vi "Autonomous Independent.vi"   [LabVIEW 2020]
doc: "This VI is called when autonomous begins, and will automatically be terminated when autonomous ends. You can carry out timed or sensor driven robot movement independently without needing to return to the caller."
uses:
  <vilib>/Rock Robotics/WPI/Utilities/WPI_GetSetVariantRefNum.vi
  <vilib>/Rock Robotics/Network Tables/NT Read String.vi
  <vilib>/Rock Robotics/Network Tables/NT Write Numeric Array.vi
  <vilib>/Rock Robotics/Network Tables/NT Write Number.vi
  <vilib>/Rock Robotics/WPI/RobotDrive/WPI_RobotDriveArcadeDrive_Standard(NoSaturation).vi
  Robot Global Data.vi
panel:
  # "Be sure to right-click and choose Data Operations>>Make Current Value default if you want to save the array values with the VI"
types:
  T1 = typedef "WPI_JoystickDevRef.ctl" = cluster{"Device":T2}
  T2 = typedef "WPI_JoystickDeviceEnum.ctl" = enum16{"USB 0", "USB 1", "USB 2", "USB 3", "USB 4", "USB 5"}
  T3 = typedef "WPI_RobotDriveDevRef.ctl" = cluster{"DevStatus":errorcluster, "Motors[]":T4[], "Square Inputs":bool, "Max Output":dbl}
  T4 = typedef "WPI_MotorControlDeviceRef.ctl" = cluster{"DeviceStatus":errorcluster, "Type":T5, "PWM":cluster{"PWM Channel":T6, "DeadBand":T7}, "CAN":cluster{"Device Number":u8, "SetOutput VI Ref":variant, "GetOutput VI Ref":variant, "Enable VI Ref":variant, "Disable VI Ref":variant, "Data":variant}, "Invert":bool, "DIO PWM":cluster{"PWM \"Enable\" Channel":T6, "DIOChannel":T8, "PWM Rate":dbl}}
  T5 = typedef "WPI_MotorControlType.ctl" = enum16{"PWM", "CAN", "DIO PWM"}
  T6 = typedef "FPGA_DIOPWMChannel.ctl" = enum8{"PWM 0", "PWM 1", "PWM 2", "PWM 3", "PWM 4", "PWM 5", "PWM 6", "PWM 7", "PWM 8", "PWM 9", "PWM MXP 0", "PWM MXP 1", "PWM MXP 2", "PWM MXP 3", "PWM MXP 4", "PWM MXP 5", "PWM MXP 6", "PWM MXP 7", "PWM MXP 8", "PWM MXP 9", "Invalid"}
  T7 = typedef "WPI_PWMDeadband.ctl" = cluster{"Name":string, "maxPositivePwm":i32, "minPositivePwm":i32, "centerPwm":i32, "maxNegativePwm":i32, "minNegativePwm":i32, "angularRange":u16}
  T8 = typedef "FPGA_DIOChannel.ctl" = enum8{"DIO 0", "DIO 1", "DIO 2", "DIO 3", "DIO 4", "DIO 5", "DIO 6", "DIO 7", "DIO 8", "DIO 9", "DIO MXP 0", "DIO MXP 1", "DIO MXP 2", "DIO MXP 3", "DIO MXP 4", "DIO MXP 5", "DIO MXP 6", "DIO MXP 7", "DIO MXP 8", "DIO MXP 9", "DIO MXP 10", "DIO MXP 11", "DIO MXP 12", "DIO MXP 13", "DIO MXP 14", "DIO MXP 15", "SPI Port CS1", "SPI Port CS2", "SPI Port CS3", "SPI Port MISO", "SPI Port MOSI", "Invalid"}
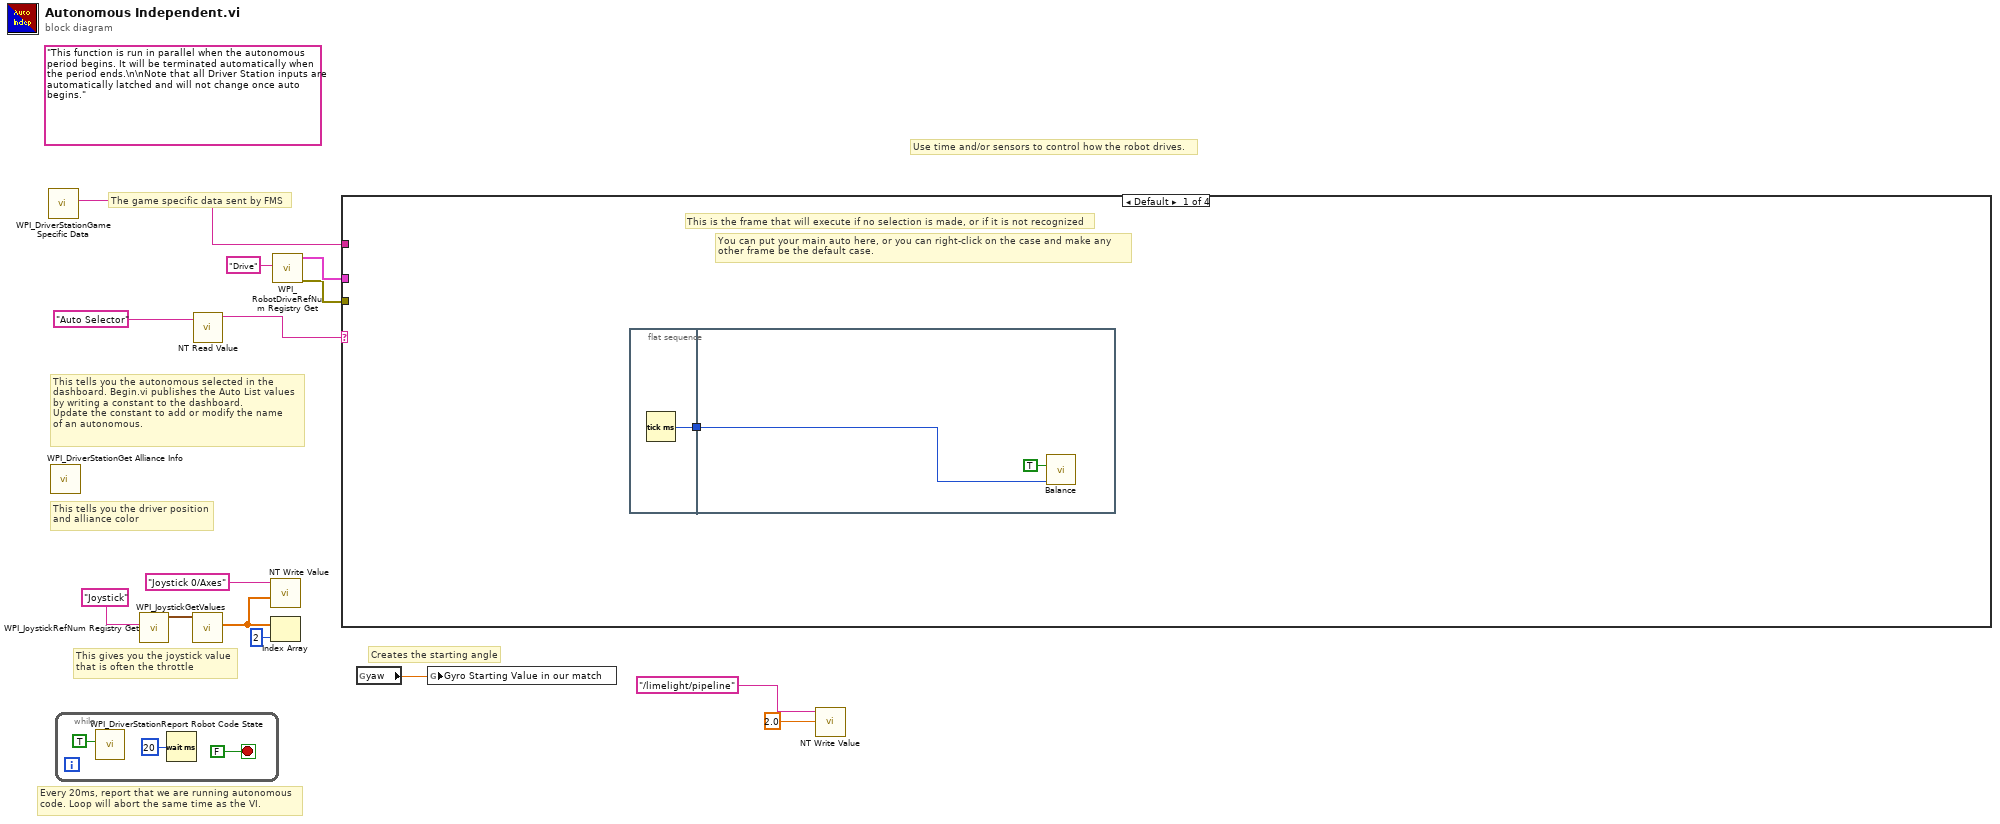
[diagram p0: block diagram]
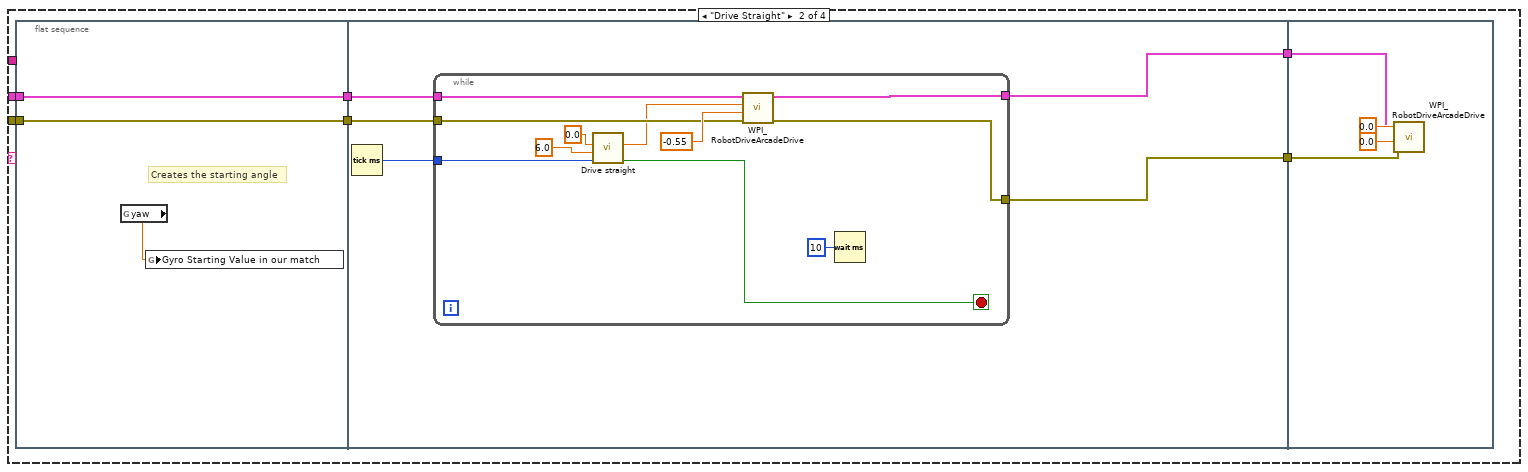
[diagram p2: hidden frame]
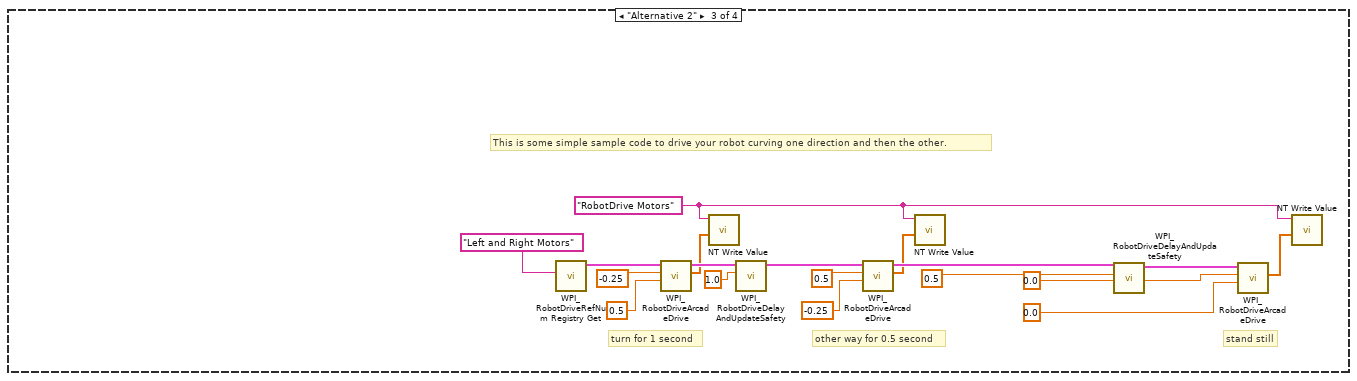
[diagram p3: hidden frame]
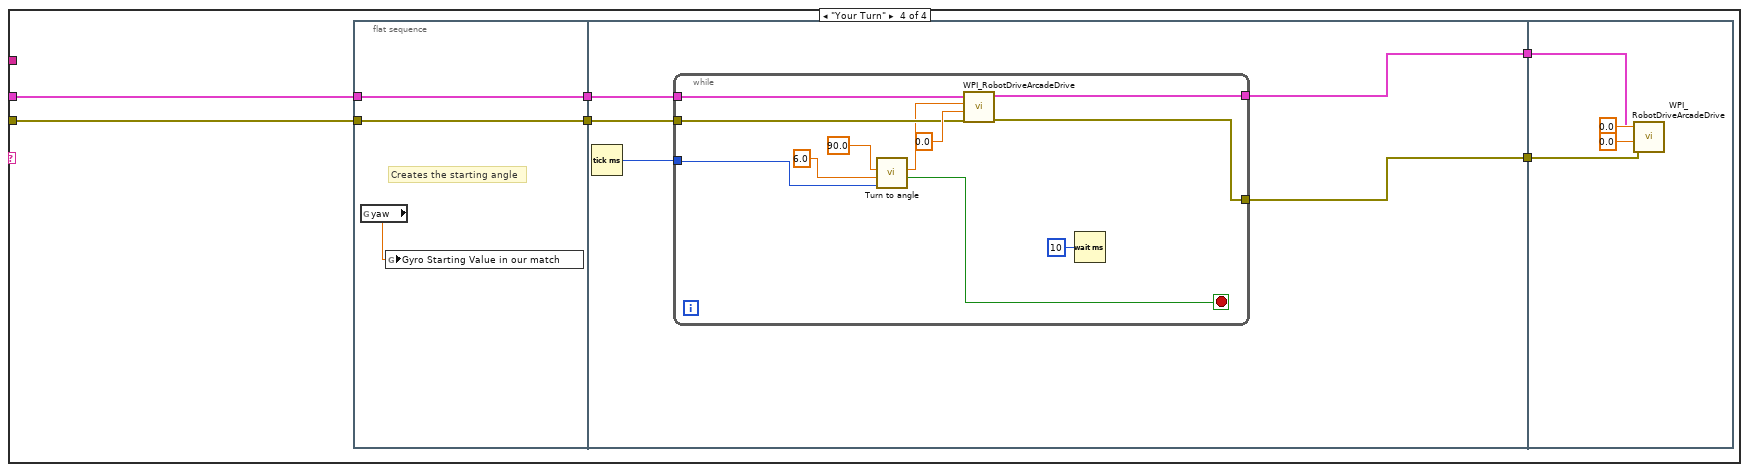
[diagram p4: hidden frame]
diagram:
  (unwired) "This function is run in parallel when the autonomous period begins. It will be terminated automatically when the period ends.\n\nNote that all Driver Station inputs are automatically latched and will not change once auto begins."
  # "Creates the starting angle"
  # "The game specific data sent by FMS"
  # "This tells you the autonomous selected in the \ndashboard. Begin.vi publishes the Auto List values\nby writing a constant to the dashboard.\nUpdate the constant to add or modify the name\nof an autonomous."
  # "Every 20ms, report that we are running autonomous\ncode. Loop will abort the same time as the VI."
  # "This gives you the joystick value\nthat is often the throttle"
  # "Use time and/or sensors to control how the robot drives."
  # "This tells you the driver position\nand alliance color"
  n1 = call <vilib>:"WPI_DriverStationGame Specific Data.vi"() -> ("Game Specific Data"=w7:string)  [unwired: 11 in]
  n2 = call <vilib>:"WPI_DriverStationGet Alliance Info.vi"() -> ()  [unwired: 12 out]
  n3 = while {
    stop <- FALSE stop-if-true
    n4 = call <vilib>:"WPI_DriverStationReport Robot Code State.vi"("Autonomous"=TRUE) -> ()  [unwired: 10 in, 1 out]
    n5 = Wait (ms)(milliseconds to wait=u32 20) -> ()  [unwired: 1 out]
  }
  n6 = call <vilib>:"WPI_JoystickRefNum Registry Get.vi"("refnum name"="Joystick") -> ("JoystickDevRef"=w13:T1)  [unwired: 1 in, 9 out]
  n7 = call <vilib>:"WPI_JoystickGetValues.vi"("JoystickDevRef"=w13) -> ("Axes"=w9:dbl[])  [unwired: 6 in, 4 out]
  n8 = call-poly <vilib>:"NT Read Value.vi"("name"="Auto Selector" ("Name")) -> ("value"=w10:string)  [unwired: 8 in, 2 out]
  n9 = call-poly <vilib>:"NT Write Value.vi"("value"=w9, "name"="Joystick 0/Axes" ("Name")) -> ()  [unwired: 9 in, 1 out]
  n10 = Index Array(array=w9, index=2) -> ()  [unwired: 1 out]
  n11 = call <vilib>:"WPI_RobotDriveRefNum Registry Get.vi"("refnum name"="Drive") -> ("error out"=w4:errorcluster, "RobotDriveDevRef"=w5:T3)  [unwired: 9 in]
  n12 = case shown="Default" w10 {
    tunnel: w7 -> [_ _ _ _]
    tunnel: w5 -> [_ w23 _ w72]
    tunnel: w4 -> [_ w22 _ w71]
    frame Default {
      # "You can put your main auto here, or you can right-click on the case and make any\nother frame be the default case."
      # "This is the frame that will execute if no selection is made, or if it is not recognized"
      n13 = flat-sequence {
        tunnel: [w19] -> w18
        tunnel: w18 -> [w21]
        frame #0 {
          n14 = Tick Count (ms)() -> (millisecond timer value=w19:u32)
        }
        frame #1 {
          n15 = call "Balance.vi"("Start Time"=w21, "Boolean"=TRUE) -> ()  [unwired: 10 in]
        }
      }
    }
    frame "Drive Straight" {
      n16 = flat-sequence {
        tunnel: w22 -> [w29]
        tunnel: w23 -> [w30]
        tunnel: [w30] -> w27
        tunnel: [w29] -> w26
        tunnel: [w35] -> w25
        tunnel: [w34] -> w24
        tunnel: w27 -> [w33]
        tunnel: w26 -> [w32]
        tunnel: w25 -> [w48]
        tunnel: w24 -> [w47]
        frame #0 {
          # "Creates the starting angle"
          n17 = global read "Robot Global Data.vi" "yaw"() -> (w28:dbl)
          n18 = global write "Robot Global Data.vi" "Gyro Starting Value in our match"(w28) -> ()
        }
        frame #1 {
          n19 = Tick Count (ms)() -> (millisecond timer value=w31:u32)
          n20 = while {
            tunnel: [w45] -> w35
            tunnel: [w44] -> w34
            tunnel: w33 -> [w43]
            tunnel: w32 -> [w41]
            tunnel: w31 -> [w40]
            stop <- w36 stop-if-true
            n21 = call "Drive straight.vi"("Start Time"=w40, "Length(seconds)"=6.0, "Desired angle"=0.0) -> ("Complete or not"=w36:bool, "X Power"=w37:dbl)  [unwired: 7 in]
            n22 = call-poly <vilib>:"WPI_RobotDriveArcadeDrive.vi"("error in (no error)"=w41, "Y axis value"=-0.55, "X axis value"=w37, "RobotDriveDevRef"=w43) -> ("error out"=w44:errorcluster, "RobotDriveDevRef"=w45:T3)  [unwired: 5 in, 1 out]
            n23 = Wait (ms)(milliseconds to wait=u32 10) -> ()  [unwired: 1 out]
          }
        }
        frame #2 {
          n24 = call-poly <vilib>:"WPI_RobotDriveArcadeDrive.vi"("error in (no error)"=w47, "Y axis value"=0.0, "X axis value"=0.0, "RobotDriveDevRef"=w48) -> ()  [unwired: 5 in, 3 out]
        }
      }
    }
    frame "Alternative 2" {
      w52 = "RobotDrive Motors" ("Name")
      # "This is some simple sample code to drive your robot curving one direction and then the other."
      # "stand still"
      # "other way for 0.5 second"
      # "turn for 1 second"
      n25 = call <vilib>:"WPI_RobotDriveRefNum Registry Get.vi"("refnum name"="Left and Right Motors") -> ("RobotDriveDevRef"=w68:T3)  [unwired: 1 in, 9 out]
      n26 = call-poly <vilib>:"WPI_RobotDriveArcadeDrive.vi"("Y axis value"=0.5 ("X axis value"), "X axis value"=-0.25, "RobotDriveDevRef"=w68) -> ("Motor Values"=w51:dbl[], "RobotDriveDevRef"=w61:T3)  [unwired: 1 in, 6 out]
      n27 = call-poly <vilib>:"NT Write Value.vi"("value"=w51, "name"=w52) -> ()  [unwired: 9 in, 1 out]
      n28 = call <vilib>:"WPI_RobotDriveDelayAndUpdateSafety.vi"("Delay (s)"=1.0, "RobotDriveDevRef"=w61) -> ("RobotDriveDevRef 2"=w62:T3)  [unwired: 8 in, 1 out]
      n29 = call-poly <vilib>:"WPI_RobotDriveArcadeDrive.vi"("Y axis value"=-0.25 ("X axis value"), "X axis value"=0.5, "RobotDriveDevRef"=w62) -> ("Motor Values"=w53:dbl[], "RobotDriveDevRef"=w63:T3)  [unwired: 1 in, 6 out]
      n30 = call-poly <vilib>:"NT Write Value.vi"("value"=w53, "name"=w52) -> ()  [unwired: 9 in, 1 out]
      n31 = call <vilib>:"WPI_RobotDriveDelayAndUpdateSafety.vi"("Delay (s)"=0.5, "RobotDriveDevRef"=w63) -> ("RobotDriveDevRef 2"=w64:T3)  [unwired: 8 in, 1 out]
      n32 = call-poly <vilib>:"WPI_RobotDriveArcadeDrive.vi"("Y axis value"=0.0 ("X axis value"), "X axis value"=0.0, "RobotDriveDevRef"=w64) -> ("Motor Values"=w54:dbl[])  [unwired: 1 in, 7 out]
      n33 = call-poly <vilib>:"NT Write Value.vi"("value"=w54, "name"=w52) -> ()  [unwired: 9 in, 1 out]
    }
    frame "Your Turn" {
      n34 = flat-sequence {
        tunnel: w71 -> [w76]
        tunnel: w72 -> [w77]
        tunnel: [w77] -> w70
        tunnel: [w76] -> w69
        tunnel: [w82] -> w74
        tunnel: [w81] -> w73
        tunnel: w70 -> [w80]
        tunnel: w69 -> [w79]
        tunnel: w74 -> [w95]
        tunnel: w73 -> [w94]
        frame #0 {
          # "Creates the starting angle"
          n35 = global read "Robot Global Data.vi" "yaw"() -> (w75:dbl)
          n36 = global write "Robot Global Data.vi" "Gyro Starting Value in our match"(w75) -> ()
        }
        frame #1 {
          n37 = Tick Count (ms)() -> (millisecond timer value=w78:u32)
          n38 = while {
            tunnel: [w92] -> w82
            tunnel: [w91] -> w81
            tunnel: w80 -> [w90]
            tunnel: w79 -> [w88]
            tunnel: w78 -> [w85]
            stop <- w83 stop-if-true
            n39 = call "Turn to angle.vi"("Start Time"=w85, "Range of accuracy"=sgl 6.0, "desired angle"=sgl 90.0) -> ("In Range?"=w83:bool, "coerced(x)"=w84:dbl)  [unwired: 7 in]
            n40 = call-poly <vilib>:"WPI_RobotDriveArcadeDrive.vi"("error in (no error)"=w88, "Y axis value"=0.0, "X axis value"=w84, "RobotDriveDevRef"=w90) -> ("error out"=w91:errorcluster, "RobotDriveDevRef"=w92:T3)  [unwired: 5 in, 1 out]
            n41 = Wait (ms)(milliseconds to wait=u32 10) -> ()  [unwired: 1 out]
          }
        }
        frame #2 {
          n42 = call-poly <vilib>:"WPI_RobotDriveArcadeDrive.vi"("error in (no error)"=w94, "Y axis value"=0.0, "X axis value"=0.0, "RobotDriveDevRef"=w95) -> ()  [unwired: 5 in, 3 out]
        }
      }
    }
  }
  n43 = global read "Robot Global Data.vi" "yaw"() -> (w3:dbl)
  n44 = global write "Robot Global Data.vi" "Gyro Starting Value in our match"(w3) -> ()
  n45 = call-poly <vilib>:"NT Write Value.vi"("value"=2.0, "name"="/limelight/pipeline" ("Name")) -> ()  [unwired: 9 in, 1 out]
